vi "to string.vi"(8 "error in":errorcluster, 11 "channel in":refnum<class "FPGA Channel.lvclass">) -> (0 "error out":errorcluster, 1 "channel data":string, 2 "identifier":string, 3 "channel out":refnum<class "FPGA Channel.lvclass">)   [LabVIEW 2015, in "FPGA Channel.lvclass"]
uses:
  FPGA Channel.lvclass
  FPGA Channel.lvclass/FPGA Channel.ctl
  Read FXP type.vi
  <vilib>/NI/Tag Bus Module Framework/channel/TBM channel.lvclass
  <vilib>/NI/Configuration Framework/serializable configuration/NISE_CEF_serializable configuration.lvclass
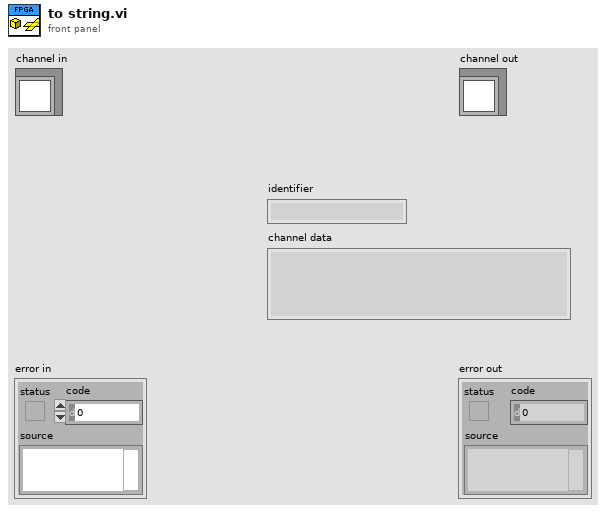
[diagram p1: front panel]
types:
  T1 = typedef "LVFixedPointRepBitsTypeDef.ctl" = cluster{"Signed":bool, "Word Length":u32, "Integer Word Length":i32}
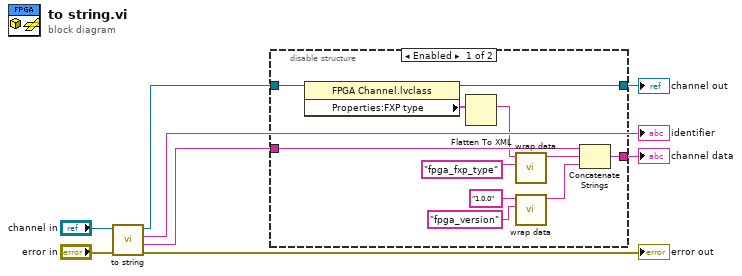
[diagram p0: block diagram]
diagram:
  n1 = call-parent "to string.vi"("error in"="error in", "channel in"="channel in") -> ("error out"=→"error out":errorcluster, "channel data"=w1:string, "identifier"=→"identifier":string, "channel out"=w4:refnum<class "FPGA Channel.lvclass">)  [unwired: 6 in]
  n2 = disable-structure shown="Enabled" {
    disable-tunnel: w4 -> [w19 w20]
    disable-tunnel: [w18 w20] -> w3
    disable-tunnel: [w13 w21] -> w2
    disable-tunnel: w1 -> [w12 w21]
    frame Enabled {
      n3 = property class="FPGA Channel.lvclass"(reference=w19) -> (reference out=w18:refnum<class "FPGA Channel.lvclass">, "Properties:FXP type"=w17:T1)  [unwired: 1 in, 1 out]
      n4 = Flatten To XML(anything=w17) -> (xml string=w10:string)
      n5 = call <vilib>:"wrap data.vi"("identifier"="fpga_fxp_type" ("additional identifier"), "data to wrap"=w10) -> ("wrapped data"=w11:string)  [unwired: 9 in]
      n6 = call <vilib>:"wrap data.vi"("identifier"="fpga_version", "data to wrap"="1.0.0") -> ("wrapped data"=w9:string)  [unwired: 9 in]
      n7 = Concatenate Strings(w12, w11, w9) -> (w13:string)
    }
    frame Disabled {
    }
  }
  "channel out" <- w3
  "channel data" <- w2
